vi "findAllyOrEnemyRobotClosestToBall.vi"(8 "error in (no error)":errorcluster, 9 "Ally/Enemy Robots":refnum<class "Robot.lvclass">[](array[class]), 10 "Ball":refnum<class "Ball.lvclass">, 11 "Utilities in":refnum<class "Utilities.lvclass">) -> (0 "error out":errorcluster, 1 "Robot distance to ball":dbl, 2 "Robot":refnum<class "Robot.lvclass">, 3 "Utilities out":refnum<class "Utilities.lvclass">)   [LabVIEW 2021, in "Utilities.lvclass"]
uses:
  Utilities.lvclass
  Robot_class/Robot.lvclass
  D:/RoboIme/horie/SSL_AI/Object_class/Object.lvclass
  Ball_class/Ball.lvclass
  Object_class/Object.lvclass/Object.ctl
  Object_class/Read x.vi
  Object_class/Read y.vi
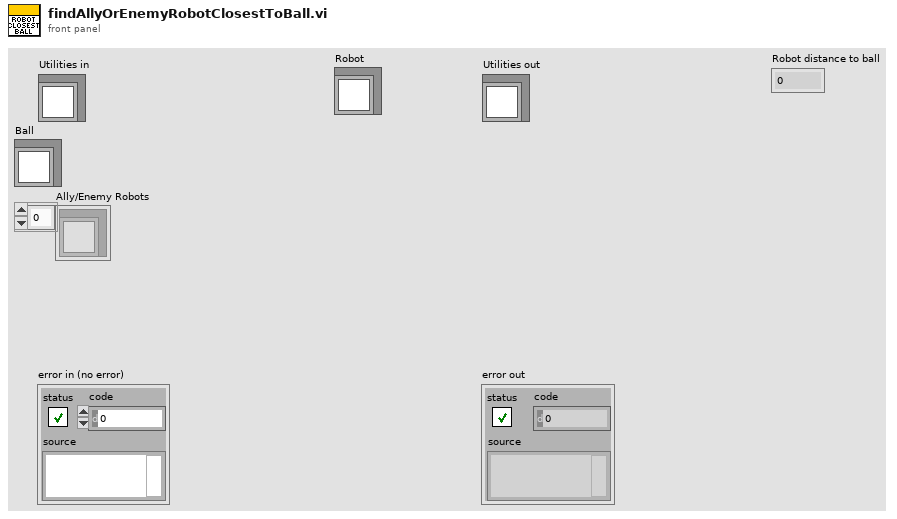
[diagram p1: front panel]
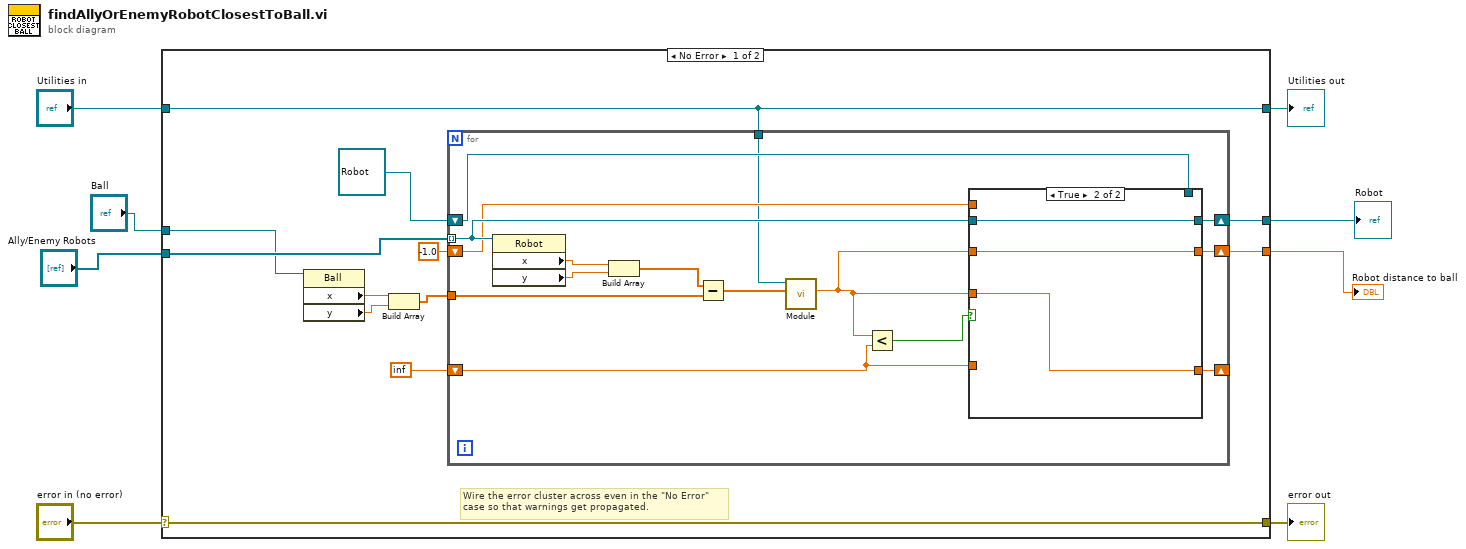
[diagram p0: block diagram]
diagram:
  n1 = case shown="No Error" "error in (no error)" {
    selector: "error in (no error)" -> [w20 w43]
    tunnel: [w20 w43] -> w7
    tunnel: [w10 w42] -> w5
    tunnel: "Utilities in" -> [w10 w42]
    tunnel: [w15 _] -> w4
    tunnel: "Ally/Enemy Robots" -> [w13 _]
    tunnel: [w12 _] -> w2
    tunnel: "Ball" -> [w9 _]
    frame No Error {
      # "Wire the error cluster across even in the \"No Error\"\ncase so that warnings get propagated."
      n2 = property class="Ball"(reference=w9) -> ("x"=w19:dbl, "y"=w18:dbl)  [unwired: 1 in, 2 out]
      n3 = Build Array(w19, w18) -> (w17:dbl[])
      n4 = for {
        tunnel: w13 -> [w26] mode=indexing
        tunnel: w17 -> [w32]
        shift-right: [w29] -> _
        shift-left: inf -> [w28]
        shift-right: [w27] -> w15
        shift-left: refnum<class "Robot.lvclass"> refnum ("Robot") -> [w25]
        shift-right: [w24] -> w12
        shift-left: -1.0 ("Modulo") -> [w22]
        tunnel: w10 -> [w21]
        n5 = property class="Robot"(reference=w26) -> ("x"=w35:dbl, "y"=w34:dbl)  [unwired: 1 in, 2 out]
        n6 = Build Array(w35, w34) -> (w33:dbl[])
        n7 = Subtract(x=w33, y=w32) -> (x-y=w31:dbl[])
        n8 = call "Module.vi"("2D vector"=w31, "Utilities in"=w21) -> ("Modulo"=w23:dbl)  [unwired: 7 in, 2 out]
        n9 = Less?(x=w23, y=w28) -> (x < y?=w30:bool)
        n10 = case shown="True" w30 {
          tunnel: [w38 w41] -> w29
          tunnel: w23 -> [_ w41]
          tunnel: w28 -> [w38 _]
          tunnel: [w37 w40] -> w27
          tunnel: w26 -> [_ w40]
          tunnel: w25 -> [w37 _]
          tunnel: [w36 w39] -> w24
          tunnel: w23 -> [_ w39]
          tunnel: w22 -> [w36 _]
          frame False {
          }
          frame True {
          }
        }
      }
    }
    frame Error {
    }
  }
  "error out" <- w7
  "Utilities out" <- w5
  "Robot" <- w4
  "Robot distance to ball" <- w2
